vi "lits unmerged vis.vi"() -> (3 "Unmerged VIs candidates":string[](array[string]))   [LabVIEW 2022 SP3]
panel:
  out "size(s)":i32
  in  "VI List":string="mini gridder/picker app/super spot find/super spot find.read write configuration.vi\nmini gridder/picking head.calculate pin offset brasil.vi\nmini gridder/picking test/TEST IMAGE PICK.vi\nmini gridder/picking test/picker.pick test no inoc colonies.vi\nmini gridder/picking test/single pin test pick.vi\nmini gridder/plate handling/lift and rotate/lift and rotate.lid up down over holder.vi\nmini gridder/plate handling/plate handling high level/plate handling.global.vi\nmini gridder/rearraying/k62 rearray dip in daughter plate end of run.vi\nmini gridder/rearraying/k62 rearray dip in daughter plate.vi\nmini gridder/rearraying/k62 rearray dip in daughter.vi\nmini gridder/rearraying/new rearraying/remote rearraying get mother plate.vi\nmini gridder/rearraying/new to bring over/rearraying new main test.vi\nmini gridder/replication/k62 replicate main.vi\nmini gridder/replication/new replicate dip im mother plate.vi\nmini gridder/replication/new replicate/dip 32 pins in daughter.vi\nmini gridder/replication/new replicate/new replicate main multiple dips.vi\nmini gridder/replication/new replicate/new replicate main.vi\nmini gridder/replication/remote replication/remote replication get mother plate.vi\nmini gridder/replication_bra/replicate colonies with carryover.vi\nmini gridder/replication_bra/replicate k6dip in daughter.vi\nmini gridder/replication_bra/replicate k6dip in mother.vi\nmini gridder/robot light/robot light.switch off on.vi\nmini gridder/scorpion1/Retrieve plate sc1.vi\nmini gridder/scorpion1/Retrieve plate sc2.vi\nmini gridder/scorpion1/get plate sc2.vi\nmini gridder/scorpion1/init scor 1 startup.vi\nmini gridder/scorpion1/init scor 2 startup.vi\nmini gridder/scorpion1/k62 send plate details to hive 2.vi\nmini gridder/scorpion1/push plate into hive 2 hotel1.vi\nmini gridder/scorpion1/scorpion 1 .init port.vi\nmini gridder/scorpion1/scorpion 1 grip open close.vi\nmini gridder/scorpion1/scorpion 1 read mode.vi\nmini gridder/scorpion1/scorpion 1 set mode.vi\nmini gridder/scorpion1/scorpion 1.read message.vi\nmini gridder/scorpion1/scorpion 2 .init port.vi\nmini gridder/scorpion1/scorpion 2 send message.vi\nmini gridder/scorpion1/scorpion 2.read message.vi\nmini gridder/scorpion1/test hive 1 only.vi\nmini gridder/scorpion1/test hives.vi\nmini gridder/sealing station/Pod 1/get plate pod1 H1.vi\nmini gridder/sealing station/Pod 1/pod 1 send message.vi\nmini gridder/sealing station/Pod 1/pod 1.read message.vi\nmini gridder/sealing station/Pod 1/prime pod1 H1.vi\nmini gridder/sealing station/confirm plates are out of hive.vi\nmini gridder/sealing station/detect plates/check plate there hive 1 hotel 2.vi\nmini gridder/sealing station/plate high level/get next plate hive 1.vi\nmini gridder/sealing station/plate high level/lid detect prompt hive 2.vi\nmini gridder/sealing station/plate high level/main high level/get next destination plate hive 2 new single inoc.vi\nmini gridder/sealing station/plate high level/main high level/get next plate run new.vi\nmini gridder/sealing station/plate high level/new hive control/Init hive 1 and 2 variables.vi\nmini gridder/sealing station/plate high level/new hive control/check hive conveyor stopped moving.vi\nmini gridder/sealing station/plate high level/new hive control/new hive 1 get plate from hotel maint.vi\nmini gridder/sealing station/plate high level/new hive control/new hive 1 get plate from hotel.vi\nmini gridder/sealing station/plate high level/new hive control/new hive 1 init startup.vi\nmini gridder/sealing station/plate high level/new hive control/new hive 1 init.vi\nmini gridder/sealing station/plate high level/new hive control/new hive 1 lock unlock plate lock.vi\nmini gridder/sealing station/plate high level/new hive control/new hive 1 move plate on conveyor.vi\nmini gridder/sealing station/plate high level/new hive control/new hive 1 move plate to front position.vi\nmini gridder/sealing station/plate high level/new hive control/new hive 1 move plate to under hotel.vi\nmini gridder/sealing station/plate high level/new hive control/new hive 1 prime hotel.vi\nmini gridder/sealing station/plate high level/new hive control/new hive 1 push plate into hotel.vi\nmini gridder/sealing station/plate high level/new hive control/new hive 1 unprime hotel.vi\nmini gridder/sealing station/plate high level/new hive control/new hive 2 get plate from hotel.vi\nmini gridder/sealing station/plate high level/new hive control/new hive 2 init startup.vi\nmini gridder/sealing station/plate high level/new hive control/new hive 2 init.vi\nmini gridder/sealing station/plate high level/new hive control/new hive 2 lock plate.vi\nmini gridder/sealing station/plate high level/new hive control/new hive 2 move plate on conveyor.vi\nmini gridder/sealing station/plate high level/new hive control/new hive 2 move plate to front position.vi\nmini gridder/sealing station/plate high level/new hive control/new hive 2 move plate to under hotel.vi\nmini gridder/sealing station/plate high level/new hive control/new hive 2 prime hotel.vi\nmini gridder/sealing station/plate high level/new hive control/new hive 2 push plate into hotel.vi\nmini gridder/sealing station/plate high level/new hive control/new hive 2 unprime hotel.vi\nmini gridder/sealing station/plate high level/new hive control/new hives global.vi\nmini gridder/sealing station/plate high level/new hive control/set hotels to load pre init.vi\nmini gridder/sealing station/plate high level/new hive control/set hotels to load.vi\nmini gridder/sealing station/plates at hotel/are plates at hive 1 hotel 1.vi\nmini gridder/sealing station/pod 2/get plate pod2.vi\nmini gridder/sealing station/pod 2/pod 2 send message.vi\nmini gridder/sealing station/pod 2/pod 2.read message.vi\nmini gridder/sealing station/scorpion1/barcode reader.init port USB scorpion 1.vi\nmini gridder/sealing station/scorpion1/check lid detection scor 1.vi\nmini gridder/sealing station/scorpion1/get plate sc1 H2.vi\nmini gridder/sealing station/scorpion1/prime hotel 2.vi\nmini gridder/sealing station/scorpion1/scorpion 1 check error status.vi\nmini gridder/sealing station/scorpion1/scorpion 1 read status.vi\nmini gridder/sealing station/scorpion1/send plate minus offset settings to scor1.vi\nmini gridder/sealing station/scorpion1/send plate settings to scor1.vi\nmini gridder/sealing station/scorpion2/barcode reader.init port USB scorpion 2.vi\nmini gridder/sealing station/scorpion2/check lid detection scor 2.vi\nmini gridder/sealing station/scorpion2/get plate sc2 H2.vi\nmini gridder/sealing station/scorpion2/prime hotel  sc2.vi\nmini gridder/sealing station/scorpion2/transfer plate foward to stop sensor SC2.vi\nmini gridder/source stacker/core/low level/source stacker/s stack wait for in position.vi\nmini gridder/source stacker/gripper arm/s arm in down pos.vi\nmini gridder/source stacker/gripper arm/s arm in up pos.vi\nmini gridder/sstack/clean up bed.vi\nmini gridder/stacker/move/stacker move to transfer position.vi\nmini gridder/sterilise/deep blower/deep blower.dry double pins.vi\nmini gridder/sterilise/new picking head/all pins up-down.vi\nmini gridder/sterilise/sonic bath/sonic bath wash.vi\nmini gridder/sterilise/sterilise high level/sterilise.global.vi\nmini gridder/system setup/system setup.read write configuration text ini format.vi\nmini gridder/system setup/system setup.read write configuration.vi\nmini gridder/transfer shuttles/destination transfer shuttle out in.vi\nmini gridder/transfer shuttles/move robot to safe tran pos.vi\nmini gridder/transfer shuttles/source transfer shuttle out in.vi\nmini gridder/user management/user managemant.login screen.vi\nmini gridder/user management/user management.add user.vi\nmini gridder/user management/user management.run global.vi\nmini gridder/uv light/uv light.close door and on.vi\nmini gridder/uv light/uv light.on off.vi\npicker (v)/Robot.Picker/vision temp/vision temp.snap.vi\npicker.main.vi\n"
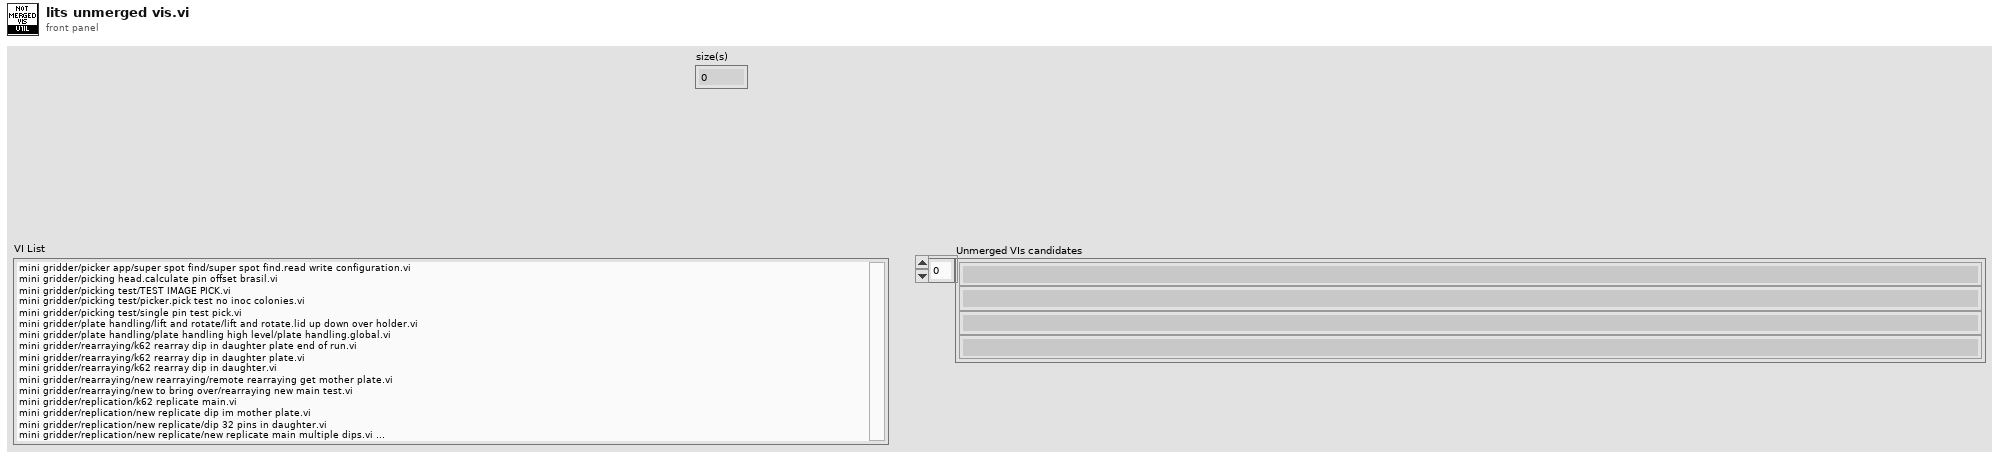
[diagram p1: front panel]
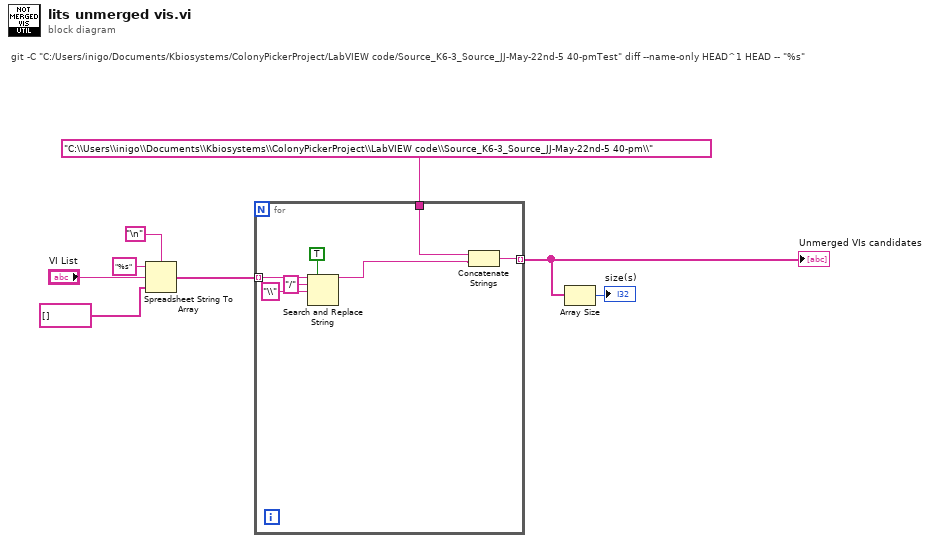
[diagram p0: block diagram]
diagram:
  # "git -C \"C:/Users/inigo/Documents/Kbiosystems/ColonyPickerProject/LabVIEW code/Source_K6-3_Source_JJ-May-22nd-5 40-pmTest\" diff --name-only HEAD^1 HEAD -- \"%s\""
  n1 = Spreadsheet String To Array(delimiter (Tab)="\n", format string="%s", spreadsheet string="VI List", array type (2D Dbl)=string[] []) -> (array=w4:string[])
  n2 = for {
    tunnel: w4 -> [w14] mode=indexing
    tunnel: [w11] -> w2 mode=indexing
    tunnel: "C:\\Users\\inigo\\Documents\\Kbiosystems\\ColonyPickerProject\\LabVIEW code\\Source_K6-3_Source_JJ-May-22nd-5 40-pm\\" -> [w10]
    n3 = Search and Replace String(replace all?=TRUE ("replace all? (F)"), input string=w14, search string="/", replace string="\\" ("replace string (\"\")")) -> (result string=w9:string)  [unwired: 4 in, 3 out]
    n4 = Concatenate Strings(w10, w9) -> (w11:string)
  }
  "Unmerged VIs candidates" <- w2
  n5 = Array Size(array=w2) -> (size(s)=→"size(s)":i32)
